vi "Who Am I.vi"(7 "I2C Channel":u8, 8 "Error In":errorcluster, 10 "I2C Slave Address (0)":u8, 11 "LINX Resource":T1) -> (0 "Error Out":errorcluster, 2 "ID":u8, 3 "LINX Resource":T1)   [LabVIEW 2011, in "LVH-LINX.lvlib" / "MMA8451.lvlib"]
doc: "Send Who Am I command to MMA8451. This command is useful to ensure the correct slave address is used and that the device is out of reset."
uses:
  MMA8451.lvlib
  Private/Type Defs/LINX Ref.ctl
  Private/Type Defs/Platform.ctl
  Private/Type Defs/Interface.ctl
  Private/Device/Type Defs/LINX Device Config.ctl
  Private/Device/Type Defs/TCP Config.ctl
  Private/Device/Type Defs/Channels.ctl
  Private/Type Defs/Peripherals/I2C/EOF.ctl
  Registers.ctl
  LVH-LINX.lvlib
  Private/Device/Device.lvlib
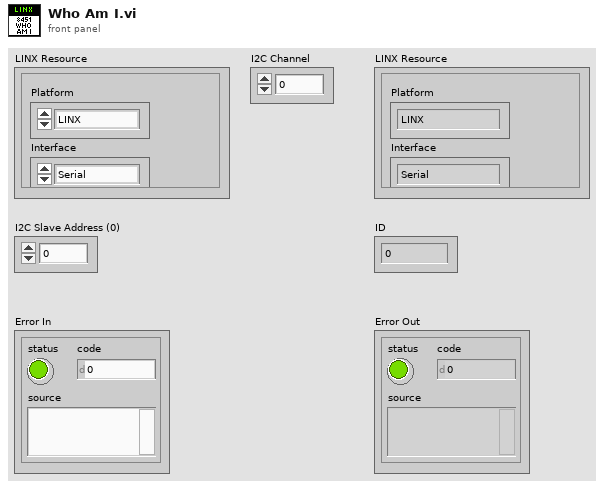
[diagram p1: front panel]
types:
  T1 = typedef "LVH-LINX.lvlib/LINX Ref.ctl" = cluster{"Platform":T2, "Interface":T3, "LINX Device Config":T4}
  T2 = typedef "LVH-LINX.lvlib/Platform.ctl" = enum16{"LINX", "myRIO"}
  T3 = typedef "LVH-LINX.lvlib/Interface.ctl" = enum16{"Serial", "TCP"}
  T4 = typedef "LVH-LINX.lvlib/Device.lvlib/LINX Device Config.ctl" = cluster{"Interface":T3, "COM Port":refnum<visa-resource-name>, "TCP Configuration":T5, "Device Family":u8, "Device ID":u8, "Device Name":string, "TCP Ref":refnum<k5>, "Channels":T6}
  T5 = typedef "LVH-LINX.lvlib/Device.lvlib/TCP Config.ctl" = cluster{"IP Address":string, "Port":u16}
  T6 = typedef "LVH-LINX.lvlib/Channels.ctl" = cluster{"DI Channels":u8[], "DO Channels":u8[], "AI":u8[], "AO":u8[], "PWM":u8[], "QE":u8[], "UART":u8[], "I2C 2":u8[], "SPI":u8[], "CAN":u8[], "AI Ref (V)":dbl, "AO Resolution (Bits)":u8, "AO Ref (V)":dbl}
  T7 = typedef "LVH-LINX.lvlib/MMA8451.lvlib/Registers.ctl" = u8
  T8 = typedef "LVH-LINX.lvlib/EOF.ctl" = enum8{"Stop", "Restart", "Restart No Stop", "No Stop"}
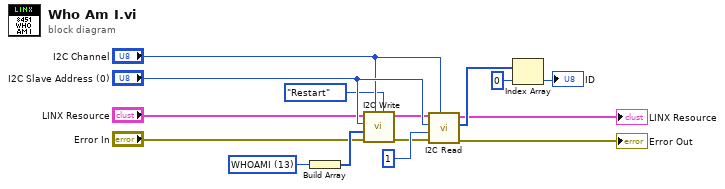
[diagram p0: block diagram]
diagram:
  w7 = T7 13 items=["OUT_X_MSB"=1, "SYSMOD"=11, "WHOAMI"=13, "XYZ_DATA_CFG"=14, "PL_STATUS"=16, "PL_CFG"=17, "CTRL_REG1"=42, "CTRL_REG2"=43, "CTRL_REG4"=45, "CTRL_REG5"=46] ("MMA8451 Register WHOAMI")
  n1 = Build Array(w7) -> (w8:T7[])
  n2 = call "I2C Write.vi"("EOF"=EOF."Restart", "I2C Channel"="I2C Channel", "Error In"="Error In", "Data"=w8, "I2C Slave Address (0)"="I2C Slave Address (0)", "LINX Resource"="LINX Resource") -> ("Error Out"=w4:errorcluster, "LINX Resource"=w5:T1)  [unwired: 4 in]
  n3 = call "I2C Read.vi"("I2C Channel"="I2C Channel", "Error In"=w4, "Bytes To Read"=u8 1, "I2C Slave Address (0)"="I2C Slave Address (0)", "LINX Resource"=w5) -> ("Error Out"=→"Error Out":errorcluster, "Data"=w13:u8[], "LINX Resource"=→"LINX Resource":T1)  [unwired: 4 in]
  n4 = Index Array(array=w13, index=0) -> (element=→"ID":u8)
